vi "Time Stamp to Dynamic Data.vi"(8 "Error In":errorcluster, 10 "Name":string, 11 "Time Stamp Control":timestamp) -> (0 "Error Out":errorcluster, 3 "Dynamic Data Type":dynamicdata(graph))   [LabVIEW 2016]
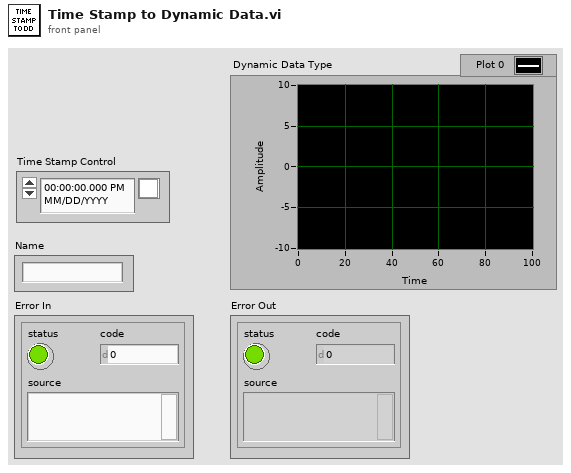
[diagram p1: front panel]
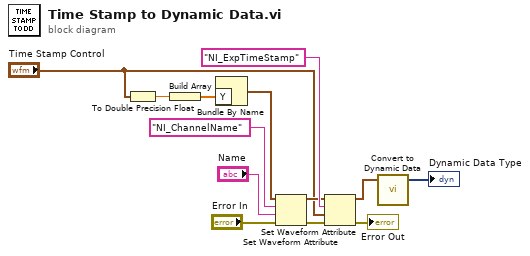
[diagram p0: block diagram]
diagram:
  n1 = To Double Precision Float(number="Time Stamp Control") -> (double precision float=w9:dbl)
  n2 = Build Array(w9) -> (w8:dbl[])
  n3 = Bundle By Name("Y"=w8) -> (w7:waveform(dbl))  [unwired: 1 in]
  n4 = Set Waveform Attribute(4:"Error In", 5:"Name", 6:"NI_ChannelName" ("name"), 7:w7) -> (0:w11:errorcluster, 3:w10:waveform(dbl))  [unwired: 1 out]
  n5 = Set Waveform Attribute(4:w11, 5:"Time Stamp Control", 6:"NI_ExpTimeStamp" ("name"), 7:w10) -> (0:→"Error Out":errorcluster, 3:w3:waveform(dbl))  [unwired: 1 out]
  n6 = call "Convert to Dynamic Data"("Waveform"=w3) -> ("Dynamic Data Type"=→"Dynamic Data Type":dynamicdata)  [unwired: 3 in]
